vi "Returning A Value Pointer To Integer Complete.vi"() -> ()   [LabVIEW 2009, in "LabVIEWWrapper_PassingDataSampleDLL.lvlib"]
uses:
  LabVIEWWrapper_PassingDataSampleDLL.lvlib
  <vilib>/Utility/importsl/GetValueByPointer/GetValueByPointer.xnode
  <vilib>/Utility/importsl/GetValueByPointer/datatype.ctl
  Program Files (x86)/National Instruments/LabVIEW 2009/resource/lvimptsl.dll
panel:
  in  "error in (no error)":errorcluster
  out "error out":errorcluster
  out "Address (Pointer)":i32
  out "Value":i32
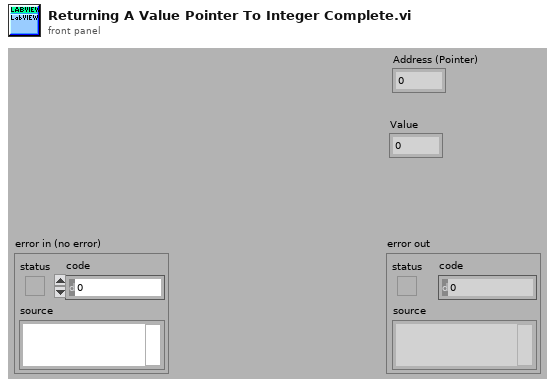
[diagram p1: front panel]
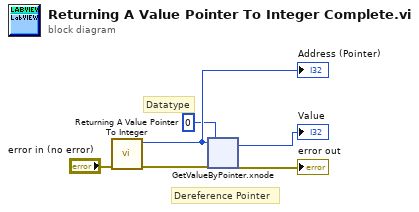
[diagram p0: block diagram]
diagram:
  # "Datatype"
  # "Dereference Pointer"
  n1 = call "Returning A Value Pointer To Integer.vi"("error in (no error)"="error in (no error)") -> ("error out"=w5:errorcluster, "function return"=w3:i32)  [unwired: 9 in]
  "Address (Pointer)" <- w3
  n2 = xnode "GetValueByPointer.xnode"("Pointer"=w3, "InputType"=0, "ErrorIn"=w5) -> ("Output"=→"Value":i32, "ErrorOut"=→"error out":errorcluster)  [unwired: 1 in]
